vi "Dashboard Main.vi"() -> ()   [LabVIEW 2020]
uses:
  <vilib>/Utility/miscctls.llb/LVRowAndColumnTypeDef.ctl
  <vilib>/event_ctls.llb/eventvkey.ctl
  <vilib>/Rock Robotics/Network Tables/NT Read Boolean.vi
  <vilib>/Rock Robotics/WPI/Dashboard/WPI_DashboardLogging Global.vi
panel:
  in  "Camera Settings Right":T1={"Frame Rate"=30, "Compression"=30, "Size"=1, "DB Camera Config"=FALSE} {"Frame Rate" scale=1.0..30.0; "Compression" scale=100.0..-1.0; "Size" items=["640x480", "320x240", "160x120"]}
  in  "Camera Name Right":string(combo)="No Camera Selection"
  out "Camera Perf":string
  in  "Camera Settings":T1={"Frame Rate"=30, "Compression"=30, "Size"=1, "DB Camera Config"=FALSE} {"Frame Rate" scale=1.0..30.0; "Compression" scale=100.0..-1.0; "Size" items=["640x480", "320x240", "160x120"]}
  in  "TCP":refnum<k5>
  in  "Rec Mode":enum32{"Stop", "Record", "Playback"}(radio)
  out "Robot IP":string
  out "Image Message":string="Timeout in Camera Communications"
  in  "Dashboard Tab":T2(tab)
  out "Grabber Motor On\nOuttake":bool
  out "Grabber Motor On\nIntake":bool
  out "Grabber Tilt Encoder R":dbl
  out "Hall Effect High":bool
  out "Hall Effect Low":bool
  out "Elevator Encoder R":dbl
  out "Elevator Encoder L":dbl
  out "Backwards Drive\nOn":bool
  out "Slow Speed\nOn":bool
  in  "Select Auto":string(combo)="Select Autonomous ..."
  out "NT Connection":bool
  out "Gyro":dbl(knob) scale=0.0..360.0
  out "Mode":T3(ring)=enum."Auto Disabled"
  out "Right Camera Perf":cluster{"Bandwidth (Mbps)":dbl, "FPS":dbl}
  out "Camera Image Right":T4(plugin-control)
  in  "DB/String 9":string
  in  "DB/String 8":string
  in  "DB/String 7":string
  in  "DB/String 6":string
  in  "DB/String 5":string
  in  "DB/String 4":string
  in  "DB/String 3":string
  in  "DB/String 2":string
  in  "DB/String 1":string
  in  "DB/String 0":string
  in  "DB/Slider 0":dbl(slide) scale=0.0..5.0
  in  "DB/Slider 1":dbl(slide) scale=0.0..5.0
  in  "DB/Slider 2":dbl(slide) scale=0.0..5.0
  in  "DB/Slider 3":dbl(slide) scale=0.0..5.0
  out "DB/LED 3":bool
  out "DB/LED 2":bool
  out "DB/LED 1":bool
  out "DB/LED 0":bool
  in  "DB/Button 3":bool
  in  "DB/Button 2":bool
  in  "DB/Button 1":bool
  in  "DB/Button 0":bool caption="New Name"
  in  "Test Slider":dbl(slide) scale=0.0..100.0 scale format="%#_3g"
  in  "On/Off":bool caption="Solenoid"
  in  "Test Name":u16(ring) items=["Select the test to run..."]
  in  "Test Tree":string(tree)
  in  "Motor":cluster{"Value":dbl, "Enable":bool} {"Value" scale=-1.0..1.0 scale format="%#_3g"}
  out "Progress":T5 {"Test Progress" scale=0.0..100.0}
  in  "Rev/Fwd":cluster{"Forward":bool, "Reverse":bool}
  in  "Test Ring":u16(ring) items=["Monochrome", "Color"]
  out "Cmd Status":string
  in  "Execute Command":bool
  in  "Command Params":string[][](table)
  in  "Command Selection":i32(listbox)
  in  "CheckList":i32(listbox)
  out "Tree":string(tree)
  out "Camera Image":T4(plugin-control)
  out "Background":bool
  in  "Camera Name":string(combo)="No Camera Selection"
  # "HW"
  # "HW"
  # "This tab is a great place for autonomous settings and robot-specific values.\nPlace controls and indicators inside this tab and match name to\nDashboard Variables on robot. You can also delete this comment."
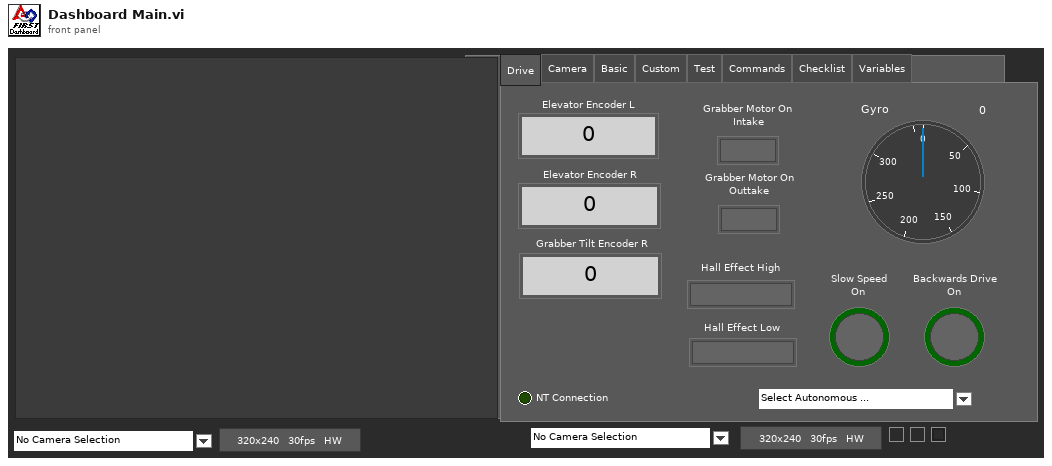
[diagram p1: front panel]
types:
  T1 = cluster{"Frame Rate":i32, "Compression":i32, "Size":u16, "DB Camera Config":bool}
  T2 = enum32{"Drive", "Camera", "Basic", "Custom", "Test", "Commands", "Checklist", "Variables"}
  T3 = enum8{"Tele-Op Disabled", "Tele-Op Enabled", "Auto Disabled", "Auto Enabled", "Test Disabled", "Test Enabled", "Disconnected", "No Code", "E-Stop"}
  T4 = typedef "IMAQ Image.ctl" = refnum<image>
  T5 = cluster{"Test Progress":u8, "Test Progress Text":string}
  T6 = cluster{"Save Path":path, "Interval (s)":dbl, "Keep":i32}
  T7 = typedef "Image Type" = u32
  T8 = cluster{"IDs":cluster{"RPC field ID":u16, "Unique ID":u16}, "String":string}
  T9 = cluster{"Error Strings":string, "Disable Counts":cluster{u16, u16}, "Rail Faults":cluster{u16, u16, u16}, "Robot IP":string, "DB Mode":u8, "Event Info":cluster{"Name":string, "Type":u8, "Number":u16, "Replay":u8}}
  T10 = cluster{"Storage":cluster{"Disk Free":u64, "RAM Block":u32, "RAM free":u32}, "CPU Utilization":cluster{"CPU % ISR":sgl, "CPU % Time Crit":sgl, "CPU % Timed Str":sgl, "CPU % High":sgl, "CPU % Above":sgl, "CPU % Normal":sgl, "CPU % Low":sgl}, "CAN":cluster{"% Bus Utilization":sgl, "Bus Off Cnt":u32, "TX_FIFO Full Cnt":u32, "Receive Error Cnt":u8, "Transmit Error Cnt":u8}, "HID":cluster{"HID Outputs":u32, "Rumble Low":u16, "Rumble High":u16}[]}
  T11 = cluster{"Status bits":cluster{"Test Mode":bool, "Autonomous":bool, "Enabled":bool, "Code Start":bool, "Brownout":bool, "Reserved 2":bool, "Reserved 3":bool, "E-Stop":bool}, "Code Trace":cluster{"Disabled":bool, "TeleOp":bool, "Auto":bool, "Test":bool}, "Controller Type":enum16{"unknown", "cRIO", "roboRio"}, "Code?":enum16{"unknown", "noCode", "code"}, "Battery V":dbl}
  T12 = cluster{"Control Bits":cluster{"TestMode":bool, "Autonomous":bool, "Enabled":bool, "FMS Present":bool, bool, bool, bool, "E-Stop":bool}, "Team Station ":u8, "Countdown":sgl, "Joystick Values":cluster{"Axes":dbl[], "Buttons":bool[], "POVs":i16[]}[]}
  T13 = cluster{"Camera Image":refnum<vi>, "Dashboard Tab":refnum<vi>, "Background":refnum<vi>, "Rec Mode":refnum<vi>, "Test Slider":refnum<vi>, "On/Off ":refnum<vi>, "Test Ring":refnum<vi>, "Rev/Fwd":refnum<vi>, "Test Name":refnum<vi>, "Motor":refnum<vi>, "Progress":refnum<vi>, "CheckList":refnum<vi>, "Tree":refnum<vi>, "Test Tree":refnum<vi>, "Command Params":refnum<vi>, "Command Selection":refnum<vi>, "Execute Command":refnum<vi>, "Cmd Status":refnum<vi>, "Camera Settings":refnum<vi>, "Camera Name":refnum<vi>, "Camera Perf":refnum<vi>, "Camera Settings Right":refnum<vi>, "Camera Name Right":refnum<vi>, "Camera Image Right":refnum<vi>}
  T14 = cluster{"Global Rectangle":i32[], "Contours":cluster{"Contour Type":u32, "ROI Type":u32, "Points":i32[]}[]}
  T15 = cluster{"Camera Name":string, string, "Saved DB Images Info":cluster{"Save Path":path, "Interval (s)":dbl, "Keep":i32}}
  T16 = cluster{"Camera Name Right":string, string, "Saved DB Images Info":cluster{"Save Path":path, "Interval (s)":dbl, "Keep":i32}}
  T17 = cluster{"Operation":enum16{"Update", "Clear"}, "Color Box":u32}[]
  T18 = typedef "eventvkey.ctl" = enum16{"ASCII", "Enter", "Return", "Shift", "Ctrl", "Alt", "Cmd", "Opt", "Caps", "NumLock", "Clear", "Break", "Up", "Down", "Left", "Right", "Insert", "Delete", "Home", "End", "PageUp", "PageDown", "Escape", "Help", "Pause", "ScrollLock", "F1", "F2", "F3", "F4", "F5", "F6", "F7", "F8", "F9", "F10", "F11", "F12", "F13", "F14", "F15", "F16", "F17", "F18", "F19", "F20", "F21", "F22", "F23", "F24", "Play", "VolumeUp", "VolumeDown", "Mute", "Two Byte Char"}
  T19 = cluster{"Image Size":bool, "Image Type":bool, "Pixel Value":bool, "ROI Information":bool, "Zoom Factor":bool}
  T20 = cluster{"Operation":enum16{"Update", "Clear"}, "Color Box":u32}
  T21 = typedef "LVRowAndColumnTypeDef.ctl" = cluster{"Row":i32, "Column":i32}
  T22 = cluster{"Shift":bool, "Ctrl":bool, "Alt":bool, "Cmd":bool, "Opt":bool}
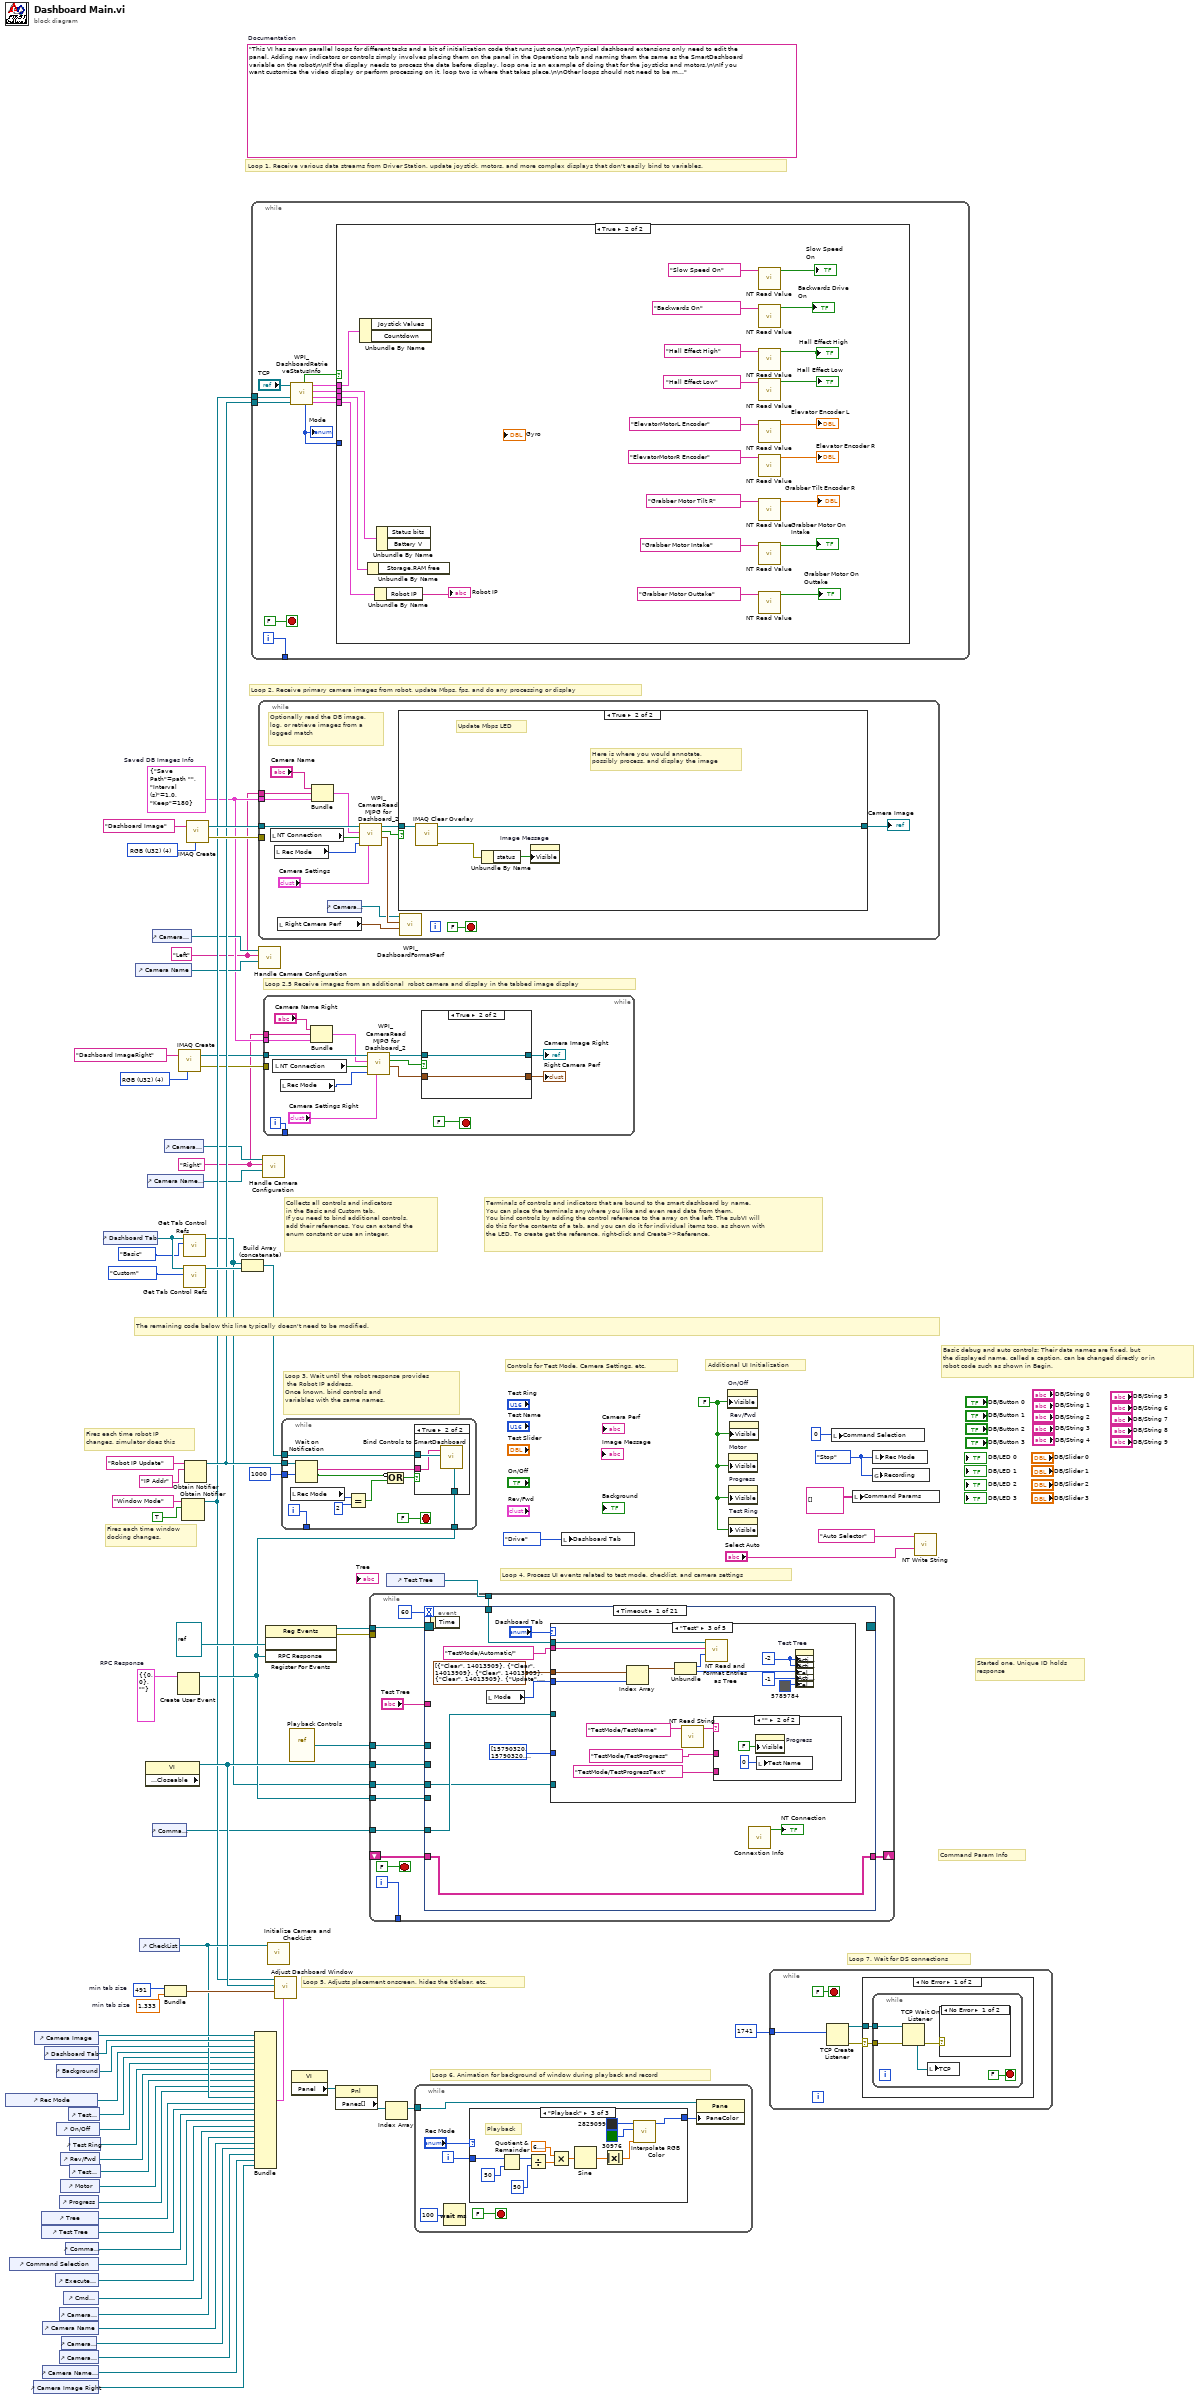
[diagram p0: block diagram]
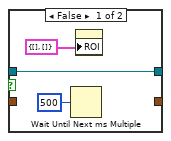
[diagram p2: hidden frame]
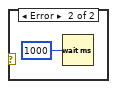
[diagram p3: hidden frame]
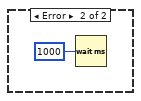
[diagram p4: hidden frame]
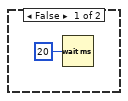
[diagram p5: hidden frame]
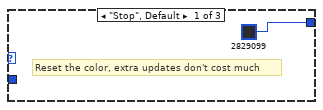
[diagram p6: hidden frame]
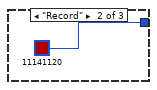
[diagram p7: hidden frame]
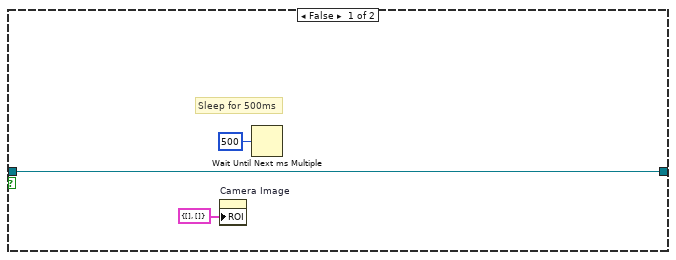
[diagram p9: hidden frame]
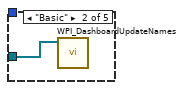
[diagram p11: hidden frame]
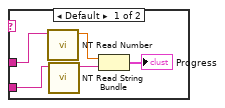
[diagram p12: hidden frame]
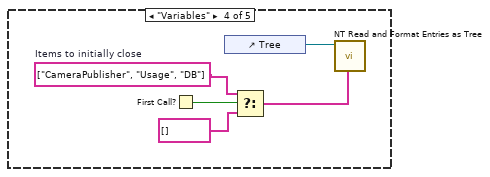
[diagram p13: hidden frame]
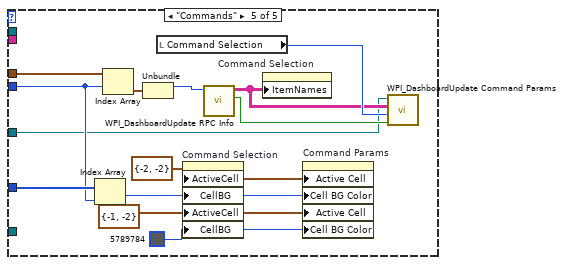
[diagram p14: hidden frame]
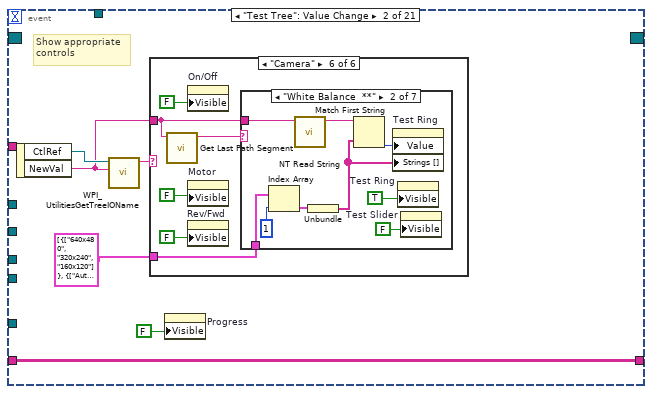
[diagram p15: hidden frame]
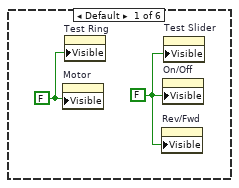
[diagram p16: hidden frame]
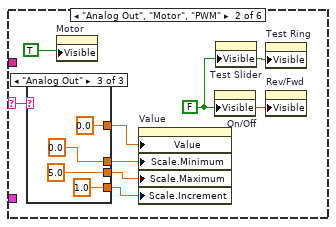
[diagram p17: hidden frame]
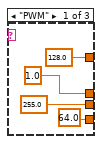
[diagram p18: hidden frame]
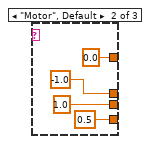
[diagram p19: hidden frame]
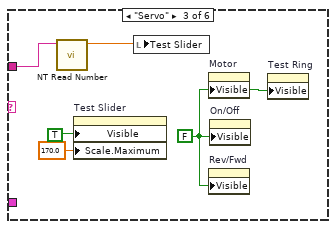
[diagram p20: hidden frame]
diagram:
  w3 = T6 {"Save Path"=path "", "Interval (s)"=1.0, "Keep"=180}  # Saved DB Images Info
  w2 = "Right"
  w1 = "Left"
  w13 = T7 4 items=["Grayscale (U8)", "Grayscale (I16)", "Grayscale (SGL)", "Complex (CSG)", "RGB (U32)", "HSL (U32)", "RGB (U64)"] ("Image Type")
  w29 = T8 {"IDs"={"RPC field ID"=0, "Unique ID"=0}, "String"=""}  # RPC Response
  w52 = 491  # min tab size
  w51 = 1.333  # min tab size
  w59 = enum32{"Stop", "Record", "Playback"}."Stop" ("Rec Mode")
  w36 = FALSE ("Visible")
  (unwired) "This VI has seven parallel loops for different tasks and a bit of initialization code that runs just once.\n\nTypical dashboard extensions only need to edit the panel. Adding new indicators or controls simply involves placing them on the panel in the Operations tab and naming them the same as the SmartDashboard variable on the robot\n\nIf the display needs to process the data before display, loop one is an example of doing that for the joysticks and motors.\n\nIf you want customize the video display or perform processing on it, loop two is where that takes place.\n\nOther loops should not need to be modified. They are pretty standard, and document the task they perform."  # Documentation
  w76 = T7 4 items=["Grayscale (U8)", "Grayscale (I16)", "Grayscale (SGL)", "Complex (CSG)", "RGB (U32)", "HSL (U32)", "RGB (U64)"] ("Image Type")
  # "Loop 2.5 Receive images from an additional  robot camera and display in the tabbed image display"
  # "Command Param Info"
  # "Started one, Unique ID holds\nresponse"
  # "Loop 7. Wait for DS connections"
  # "Basic debug and auto controls: Their data names are fixed, but\nthe displayed name, called a caption, can be changed directly or in\nrobot code such as shown in Begin."
  # "Controls for Test Mode, Camera Settings, etc."
  # "Additional UI Initialization"
  # "Loop 6. Animation for background of window during playback and record"
  # "Fires each time robot IP\nchanges, simulator does this"
  # "Fires each time window\ndocking changes."
  # "Collects all controls and indicators\nin the Basic and Custom tab.\nIf you need to bind additional controls,\nadd their references. You can extend the\nenum constant or use an integer."
  # "The remaining code below this line typically doesn't need to be modified."
  # "Loop 4. Process UI events related to test mode, checklist, and camera settings"
  # "Terminals of controls and indicators that are bound to the smart dashboard by name.\nYou can place the terminals anywhere you like and even read data from them.\nYou bind controls by adding the control reference to the array on the left. The subVI will\ndo this for the contents of a tab, and you can do it for individual items too, as shown with\nthe LED. To create get the reference, right-click and Create>>Reference."
  # "Loop 3. Wait until the robot response provides\n the Robot IP address.\nOnce known, bind controls and\nvariables with the same names."
  # "Loop 5. Adjusts placement onscreen, hides the titlebar, etc."
  # "Loop 1. Receive various data streams from Driver Station, update joystick, motors, and more complex displays that don't easily bind to variables."
  # "Loop 2. Receive primary camera images from robot, update Mbps, fps, and do any processing or display"
  n1 = control-ref of="Rec Mode"() -> (w42:refnum<vi>)
  n2 = control-ref of="Command Selection"() -> (w28:refnum<vi>)
  n3 = control-ref of="Camera Image Right"() -> (w6:refnum<vi>)
  n4 = control-ref of="Camera Image"() -> (w54:refnum<vi>)
  n5 = control-ref of="Tree"() -> (w46:refnum<vi>)
  n6 = control-ref of="Test Tree"() -> (w45:refnum<vi>)
  n7 = control-ref of="Camera Name"() -> (w19:refnum<vi>)
  n8 = control-ref of="Camera Name Right"() -> (w7:refnum<vi>)
  n9 = control-ref of="Dashboard Tab"() -> (w53:refnum<vi>)
  n10 = control-ref of="Execute Command"() -> (w30:refnum<vi>)
  n11 = control-ref of="Background"() -> (w49:refnum<vi>)
  n12 = control-ref of="On/Off"() -> (w40:refnum<vi>)
  n13 = control-ref of="Progress"() -> (w37:refnum<vi>)
  n14 = control-ref of="Camera Settings"() -> (w20:refnum<vi>)
  n15 = control-ref of="Camera Settings Right"() -> (w8:refnum<vi>)
  n16 = control-ref of="Rev/Fwd"() -> (w38:refnum<vi>)
  n17 = control-ref of="Motor"() -> (w43:refnum<vi>)
  n18 = control-ref of="Camera Perf"() -> (w18:refnum<vi>)
  n19 = control-ref of="Cmd Status"() -> (w24:refnum<vi>)
  n20 = control-ref of="Command Params"() -> (w31:refnum<vi>)
  n21 = control-ref of="Test Slider"() -> (w41:refnum<vi>)
  n22 = control-ref of="Test Ring"() -> (w39:refnum<vi>)
  n23 = control-ref of="Test Name"() -> (w44:refnum<vi>)
  n24 = control-ref of="Dashboard Tab"() -> (w57:refnum<vi>)
  n25 = control-ref of="Camera Name"() -> (w21:refnum<vi>)
  n26 = control-ref of="CheckList"() -> (w47:refnum<vi>)
  n27 = property class="VI" props=["Front Panel.Closeable"]() -> (reference out=w58:refnum<vi>)  [unwired: 2 in, 2 out]
  n28 = control-ref of="Camera Name Right"() -> (w9:refnum<vi>)
  n29 = control-ref of="Camera Settings"() -> (w22:refnum<vi>)
  n30 = control-ref of="Command Params"() -> (w23:refnum<vi>)
  n31 = control-ref of="Camera Settings Right"() -> (w10:refnum<vi>)
  n32 = Bundle("min tab size"=w52, "min tab size"=w51) -> (w50:cluster{"min tab size":i32, "min tab size":dbl})  [unwired: 1 in]
  n33 = Create User Event(user event datatype=w29) -> (user event=w25:refnum<user-event>)  [unwired: 1 in, 1 out]
  n34 = call "IMAQ Create"("Image Name"="Dashboard ImageRight", "Image Type"=w13) -> ("New Image"=w12:T4, "error out"=w11:errorcluster)  [unwired: 2 in, 1 out]
  n35 = Obtain Notifier(name (unnamed)="Window Mode", notification data type=TRUE) -> (notifier out=w34:refnum<notifier>)  [unwired: 2 in, 2 out]
  n36 = call <vilib>:"Get Tab Control Refs.vi"("Page Index"=T2."Basic" ("Dashboard Tab"), "TabControl in"=w57) -> ("ControlsOnPage"=w17:refnum<vi>[])  [unwired: 9 in]
  n37 = call <vilib>:"Get Tab Control Refs.vi"("Page Index"=T2."Custom" ("Dashboard Tab"), "TabControl in"=w57) -> ("ControlsOnPage"=w56:refnum<vi>[])  [unwired: 9 in]
  n38 = Obtain Notifier(name (unnamed)="Robot IP Update", notification data type="IP Addr" ("name (unnamed)")) -> (notifier out=w35:refnum<notifier>)  [unwired: 2 in, 2 out]
  n39 = call "IMAQ Create"("Image Name"="Dashboard Image", "Image Type"=w76) -> ("New Image"=w74:T4, "error out"=w73:errorcluster)  [unwired: 2 in, 1 out]
  n40 = Build Array (concatenate)(w17, w56) -> (w55:refnum<vi>[])
  n41 = while {
    tunnel: [w86] -> _
    tunnel: w35 -> [w80]
    tunnel: w34 -> [w77]
    i -> [w86]
    stop <- FALSE stop-if-true
    n42 = call <vilib>:"WPI_DashboardRetrieveStatusInfo.vi"("Binding Refnum"=w80, "Window Mode Notifier"=w77, "TCP Cnx"="TCP") -> ("Power and Errors"=w81:T9, "Robot Metrics"=w84:T10, "Status Info"=w85:T11, "Control Info"=w82:T12, "Robot Mode"=w79:T3, "Process?"=w83:bool)  [unwired: 3 in]
    "Mode" <- w79
    n43 = case shown="True" w83 {
      tunnel: w85 -> [_ w111]
      tunnel: w84 -> [_ w110]
      tunnel: w82 -> [_ w109]
      tunnel: w81 -> [_ w108]
      tunnel: w79 -> [_ _]
      frame False {
        n44 = Wait (ms)(milliseconds to wait=u32 20) -> ()  [unwired: 1 out]
      }
      frame True {
        n45 = Unbundle By Name(w109) -> ()  [unwired: 2 out]
        n46 = Unbundle By Name(w110) -> ()  [unwired: 1 out]
        n47 = Unbundle By Name(w108) -> ("Robot IP"=→"Robot IP":string)
        n48 = Unbundle By Name(w111) -> ()  [unwired: 2 out]
        n49 = call-poly <vilib>:"NT Read Value.vi"("Name"="Slow Speed On") -> ("Boolean"=→"Slow Speed\nOn":bool)  [unwired: 9 in, 1 out]
        n50 = call-poly <vilib>:"NT Read Value.vi"("Name"="Backwards On") -> ("Boolean"=→"Backwards Drive\nOn":bool)  [unwired: 9 in, 1 out]
        n51 = call-poly <vilib>:"NT Read Value.vi"("Name"="Hall Effect High") -> ("Boolean"=→"Hall Effect High":bool)  [unwired: 9 in, 1 out]
        n52 = call-poly <vilib>:"NT Read Value.vi"("Name"="Hall Effect Low") -> ("Boolean"=→"Hall Effect Low":bool)  [unwired: 9 in, 1 out]
        n53 = call-poly <vilib>:"NT Read Value.vi"("Name"="ElevatorMotorL Encoder") -> ("Numeric"=→"Elevator Encoder L":dbl)  [unwired: 9 in, 1 out]
        n54 = call-poly <vilib>:"NT Read Value.vi"("Name"="ElevatorMotorR Encoder") -> ("Numeric"=→"Elevator Encoder R":dbl)  [unwired: 9 in, 1 out]
        n55 = call-poly <vilib>:"NT Read Value.vi"("Name"="Grabber Motor Tilt R") -> ("Numeric"=→"Grabber Tilt Encoder R":dbl)  [unwired: 9 in, 1 out]
        n56 = call-poly <vilib>:"NT Read Value.vi"("Name"="Grabber Motor Intake") -> ("Boolean"=→"Grabber Motor On\nIntake":bool)  [unwired: 9 in, 1 out]
        n57 = call-poly <vilib>:"NT Read Value.vi"("Name"="Grabber Motor Outtake") -> ("Boolean"=→"Grabber Motor On\nOuttake":bool)  [unwired: 9 in, 1 out]
      }
    }
  }
  n58 = Bundle("Camera Image"=w54, "Dashboard Tab"=w53, "Background"=w49, "Rec Mode"=w42, "Test Slider"=w41, "On/Off"=w40, "Test Ring"=w39, "Rev/Fwd"=w38, "Test Name"=w44, "Motor"=w43, "Progress"=w37, "CheckList"=w47, "Tree"=w46, "Test Tree"=w45, "Command Params"=w31, "Command Selection"=w28, "Execute Command"=w30, "Cmd Status"=w24, "Camera Settings"=w20, "Camera Name"=w19, "Camera Perf"=w18, "Camera Settings Right"=w8, "Camera Name Right"=w7, "Camera Image Right"=w6) -> (w48:T13)  [unwired: 1 in]
  n59 = call "Handle Camera Configuration.vi"("CameraNameRef"=w21, "Display Name"=w1, "ClusterRef"=w22) -> ()  [unwired: 9 in]
  n60 = while {
    tunnel: w74 -> [w125]
    tunnel: w73 -> [_]
    tunnel: w3 -> [w118]
    tunnel: w1 -> [w115]
    stop <- FALSE stop-if-true
    # "Optionally read the DB image,\nlog, or retrieve images from a\nlogged match"
    n61 = local read "NT Connection"() -> (w119:bool)
    n62 = local read "Rec Mode"() -> (w122:enum32{"Stop", "Record", "Playback"})
    n63 = local read "Right Camera Perf"() -> (w113:cluster{"Bandwidth (Mbps)":dbl, "FPS":dbl})
    n64 = Bundle("Camera Name"="Camera Name", w115, "Saved DB Images Info"=w118) -> (w117:T15)  [unwired: 1 in]
    n65 = control-ref of="Camera Perf"() -> (w112:refnum<vi>)
    n66 = call <vilib>:"WPI_CameraRead MJPG for Dashboard_2.vi"("Camera Settings"="Camera Settings", "Rec Mode"=w122, "NT Connection"=w119, "Capture Info"=w117, "Image in"=w125) -> ("perf info"=w114:cluster{"Bandwidth (Mbps)":dbl, "fps":dbl}, "Active"=w123:bool, "Image\\ out"=w124:T4)  [unwired: 4 in]
    n67 = case shown="True" w123 {
      tunnel: w124 -> [w128 w131]
      tunnel: [w128 w130] -> w120
      frame False {
        # "Sleep for 500ms"
        n68 = property on="Camera Image" class="ImageControl"("ROI"=T14 {"Global Rectangle"=[], "Contours"=[]}) -> ()  [unwired: 2 in, 2 out]
        n69 = Wait Until Next ms Multiple(millisecond multiple=u32 500) -> ()  [unwired: 1 out]
      }
      frame True {
        # "Here is where you would annotate,\npossibly process, and display the image"
        # "Update Mbps LED"
        n70 = call "IMAQ Clear Overlay"("Image"=w131) -> ("error out"=w132:errorcluster, "Image Out"=w130:T4)  [unwired: 2 in, 7 out]
        n71 = Unbundle By Name(w132) -> ("status"=w133:bool)
        n72 = property on="Image Message" class="Str"("Visible"=w133) -> ()  [unwired: 2 in, 2 out]
      }
    }
    "Camera Image" <- w120
    n73 = call <vilib>:"WPI_DashboardFormatPerf.vi"("Right Camera Perf"=w113, "Performance"=w114, "String in"=w112) -> ()  [unwired: 9 in]
  }
  n74 = call "Handle Camera Configuration.vi"("CameraNameRef"=w9, "Display Name"=w2, "ClusterRef"=w10) -> ()  [unwired: 9 in]
  n75 = while {
    tunnel: w12 -> [w148]
    tunnel: w11 -> [_]
    tunnel: [w143] -> _
    tunnel: w3 -> [w139]
    tunnel: w2 -> [w136]
    i -> [w143]
    stop <- FALSE stop-if-true
    n76 = local read "NT Connection"() -> (w140:bool)
    n77 = local read "Rec Mode"() -> (w147:enum32{"Stop", "Record", "Playback"})
    n78 = Bundle("Camera Name Right"="Camera Name Right", w136, "Saved DB Images Info"=w139) -> (w138:T16)  [unwired: 1 in]
    n79 = call <vilib>:"WPI_CameraRead MJPG for Dashboard_2.vi"("Camera Settings"="Camera Settings Right", "Rec Mode"=w147, "NT Connection"=w140, "Capture Info"=w138, "Image in"=w148) -> ("perf info"=w134:cluster{"Bandwidth (Mbps)":dbl, "fps":dbl}, "Active"=w142:bool, "Image\\ out"=w145:T4)  [unwired: 4 in]
    n80 = case shown="True" w142 {
      tunnel: w145 -> [w150 w153]
      tunnel: [w150 w153] -> w141
      tunnel: [_ w152] -> w135
      tunnel: w134 -> [_ w152]
      frame False {
        n81 = Wait Until Next ms Multiple(millisecond multiple=u32 500) -> ()  [unwired: 1 out]
        n82 = property on="Camera Image Right" class="ImageControl"("ROI"=T14 {"Global Rectangle"=[], "Contours"=[]}) -> ()  [unwired: 2 in, 2 out]
      }
      frame True {
      }
    }
    "Camera Image Right" <- w141
    "Right Camera Perf" <- w135
  }
  n83 = register-events(refnum<vi> refnum, w25) -> (reference out=w63:refnum<event-registration>, error out=w62:errorcluster)  [unwired: 2 in]
  n84 = call "Initialize Camera and CheckList.vi"("ListBox in"=w47) -> ()  [unwired: 11 in]
  n85 = call "Adjust Dashboard Window.vi"("Sizing Refnums"=w48, "Size Constraints"=w50, "VI"=w58, "WIn Mode"=w34) -> ()  [unwired: 8 in]
  n86 = while {
    tunnel: w55 -> [w165]
    tunnel: w35 -> [w163]
    tunnel: [w161] -> _
    tunnel: u32 1000 ("milliseconds to wait") -> [w160]
    tunnel: w25 -> [w154]
    i -> [w161]
    stop <- FALSE stop-if-true
    n87 = local read "Rec Mode"() -> (w156:enum32{"Stop", "Record", "Playback"})
    n88 = Wait on Notification(notifier=w163, timeout in ms (-1)=w160) -> (notification=w162:string, timed out?=w158:bool)  [unwired: 2 in, 2 out]
    n89 = Equal?(x=w156, y=u16 2 ("Rec Mode")) -> (x = y?=w157:bool)
    n90 = Compound Arithmetic op=OR(invert w158, w157) -> (w159:bool)
    n91 = case shown="True" w159 {
      tunnel: w165 -> [_ w168]
      tunnel: w162 -> [_ w167]
      tunnel: w154 -> [_ w166]
      frame False {
      }
      frame True {
        n92 = call <vilib>:"Bind Controls to SmartDashboard.vi"("RPC ref"=w166, "Bound Control Refs"=w168, "Server IP Address"=w167) -> ()  [unwired: 9 in]
      }
    }
  }
  n93 = vi-ref "Playback Controls.vi"() -> (w64:refnum<vi>)
  n94 = property class="VI"() -> ("Panel"=w66:refnum<vi>)  [unwired: 2 in, 2 out]
  n95 = property class="Pnl"(reference=w66) -> ("Panes[]"=w67:refnum<vi>[])  [unwired: 1 in, 2 out]
  n96 = Index Array(array=w67) -> (element=w65:refnum<vi>)  [unwired: 1 in]
  n97 = control-ref of="Test Tree"() -> (w68:refnum<vi>)
  n98 = while {
    tunnel: [w178] -> _
    tunnel: w68 -> [w177]
    tunnel: w64 -> [w176]
    tunnel: w63 -> [w175]
    tunnel: w62 -> [_]
    tunnel: w58 -> [w174]
    tunnel: w25 -> [w173]
    tunnel: w23 -> [w172]
    shift-right: [w171] -> _
    shift-left: _ -> [w170]
    tunnel: w17 -> [w169]
    i -> [w178]
    stop <- FALSE stop-if-true
    n99 = event shown="[0] Timeout" {
      selector: w175 -> [_ _ _ _ _ _ _ _ _ _ _ _ _ _ _ _ _ _ _ _ _]
      dyn-events: [_ _ _ _ _ _ _ _ _ _ _ _ _ _ _ _ w438 _ _ _ _] -> _
      timeout: u32 60 ("milliseconds to wait") -> [_ _ _ _ _ _ _ _ _ _ _ _ _ _ _ _ _ _ _ _ _]
      tunnel: w177 -> [w190 _ _ _ _ _ _ _ _ _ _ _ _ _ _ _ _ _ _ _ _]
      tunnel: "Test Tree" -> [_ _ _ _ _ _ _ _ _ _ _ w405 w413 w415 w419 w427 _ _ _ _ _]
      tunnel: w176 -> [_ _ _ _ _ _ _ _ _ _ _ _ _ _ _ _ w440 _ w458 _ _]
      tunnel: w174 -> [_ _ _ _ _ _ _ _ _ _ _ _ _ _ _ _ w436 _ _ _ _]
      tunnel: w173 -> [_ _ _ _ _ _ _ _ _ _ _ _ _ _ _ _ w434 _ _ _ _]
      tunnel: w172 -> [w185 _ _ _ _ _ w356 _ _ _ _ _ _ _ _ _ _ _ _ _ _]
      tunnel: [w184 w233 w335 w340 w349 w353 w354 w363 w373 w380 w392 w404 w411 w414 w418 w426 w433 w453 w455 w459 w472] -> w171
      tunnel: w170 -> [w184 w233 w335 w340 w349 w353 w354 _ _ w380 w392 w404 w411 w414 w418 w426 w433 w453 w455 w459 w472]
      tunnel: w169 -> [w182 _ _ _ _ _ _ _ _ _ _ _ _ _ _ _ _ _ _ _ _]
      event Timeout {
        n100 = event-data() -> ()  [unwired: 1 in, 1 out]
        n101 = local read "Mode"() -> (w187:T3)
        n102 = case shown="\"Test\"" "Dashboard Tab" {
          tunnel: w190 -> [_ _ w206 _ _]
          tunnel: "TestMode/Automatic/" ("Name Pattern") -> [_ _ w205 _ _]
          tunnel: T17 [{"Operation"=enum."Clear", "Color Box"=14013909}, {"Operation"=enum."Clear", "Color Box"=14013909}, {"Operation"=enum."Clear", "Color Box"=14013909}, {"Operation"=enum."Clear", "Color Box"=14013909}, {"Operation"=enum."Update", "Color Box"=14013909}, {"Operation"=enum."Update", "Color Box"=16777215}, {"Operation"=enum."Clear", "Color Box"=14013909}, {"Operation"=enum."Clear", "Color Box"=14013909}, {"Operation"=enum."Clear", "Color Box"=14013909}] -> [_ _ w198 _ w226]
          tunnel: w187 -> [_ _ w197 _ w225]
          tunnel: u32[] [15790320, 15790320, 15790320, 15790320, 16777215, 16777215, 15790320, 15790320, 15790320] -> [_ _ _ _ w231]
          tunnel: w185 -> [_ _ _ _ w219]
          tunnel: w182 -> [_ w192 _ _ _]
          frame "Custom", Default {
          }
          frame "Basic" {
            n103 = call <vilib>:"WPI_DashboardUpdateNames.vi"("Controls on Tab"=w192) -> ()  [unwired: 11 in]
          }
          frame "Test" {
            w204 = -2 ("Active Item:Row Number")
            n104 = Index Array(array=w198, index=w197) -> (element=w199:T20)
            n105 = Unbundle(w199) -> ("Operation"=w200:enum16{"Update", "Clear"}, "Color Box"=w201:u32)
            n106 = call <vilib>:"NT Read String.vi"("Name"="TestMode/TestName") -> ("String"=w195:string)  [unwired: 9 in, 1 out]
            n107 = call <vilib>:"NT Read and Format Entries as Tree.vi"("Operation"=w200, "Name Pattern"=w205, "Tree Refnum"=w206) -> ()  [unwired: 7 in, 2 out]
            n108 = case shown="\"\"" w195 {
              tunnel: "TestMode/TestProgress" ("Name") -> [w208 _]
              tunnel: "TestMode/TestProgressText" ("Name") -> [w207 _]
              frame Default {
                n109 = call <vilib>:"NT Read Number.vi"("Name"=w208) -> ("Numeric"=w209:dbl)  [unwired: 9 in, 1 out]
                n110 = call <vilib>:"NT Read String.vi"("Name"=w207) -> ("String"=w210:string)  [unwired: 9 in, 1 out]
                n111 = Bundle("Numeric"=w209, "String"=w210) -> (→"Progress":cluster{"Numeric":dbl, "String":string})  [unwired: 1 in]
              }
              frame "" {
                n112 = property on="Progress" class="Clust (strict)"("Visible"=FALSE) -> ()  [unwired: 2 in, 2 out]
                n113 = local write "Test Name"(u16 0) -> ()
              }
            }
            n114 = property on="Test Tree" class="Tree (strict)"("Active Item Row Number"=w204, "ActiveColNum"=w204, "CellBG"=w201, "Active Item Row Number"=-1 ("Active Item:Row Number"), "CellBG"=u32 5789784 ("Color Box")) -> ()  [unwired: 2 in, 2 out]
          }
          frame "Variables" {
            w216 = string[] ["CameraPublisher", "Usage", "DB"]  # Items to initially close
            n115 = First Call?() -> (First Call?: T/F=w217:bool)
            n116 = control-ref of="Tree"() -> (w218:refnum<vi>)
            n117 = Select(t=w216, s=w217, f=string[] []) -> (s? t:f=w214:string[])
            n118 = call <vilib>:"NT Read and Format Entries as Tree.vi"("Tags to  Close"=w214, "Tree Refnum"=w218) -> ()  [unwired: 8 in, 2 out]
          }
          frame "Commands" {
            w227 = u32 5789784 ("Color Box")
            w228 = T21 {"Row"=-1, "Column"=-2} ("Active Cell:Active Cell")
            w230 = T21 {"Row"=-2, "Column"=-2} ("Active Cell:Active Cell")
            n119 = Index Array(array=w231, index=w225) -> (element=w229:u32)
            n120 = Index Array(array=w226, index=w225) -> (element=w224:T20)
            n121 = Unbundle(w224) -> ("Operation"=w223:enum16{"Update", "Clear"})  [unwired: 1 out]
            n122 = local read "Command Selection"() -> (w222:i32)
            n123 = property on="Command Selection" class="MCListbox (strict)"("ActiveCell"=w230, "CellBG"=w229, "ActiveCell"=w228, "CellBG"=w227) -> ()  [unwired: 2 in, 2 out]
            n124 = call <vilib>:"WPI_DashboardUpdate RPC Info.vi"("Operation"=w223) -> ("update"=w221:bool, "commands"=w220:string[][])  [unwired: 9 in]
            n125 = property on="Command Selection" class="MCListbox (strict)"("ItemNames"=w220) -> ()  [unwired: 2 in, 2 out]
            n126 = property on="Command Params" class="Tbl (strict)"("Active Cell"=w230, "Cell BG Color"=w229, "Active Cell"=w228, "Cell BG Color"=w227) -> ()  [unwired: 2 in, 2 out]
            n127 = call <vilib>:"WPI_DashboardUpdate Command Params.vi"("Update"=w221, "NewVal"=w222, "Commands"=w220, "Param Tbl"=w219) -> ()  [unwired: 7 in, 1 out]
          }
        }
        n128 = call <vilib>:"Connextion Info.vi"() -> ("Connected"=→"NT Connection":bool)  [unwired: 10 in, 1 out]
      }
      event "Test Tree": Value Change {
        # "Show appropriate\ncontrols"
        n129 = event-data() -> ("CtlRef"=w236:refnum<vi>, "NewVal"=w234:string)  [unwired: 1 in]
        n130 = call <vilib>:"WPI_UtilitiesGetTreeIOName.vi"("NewVal"=w234, "TreeControl in"=w236) -> ("I/O Name"=w237:string)  [unwired: 9 in]
        n131 = case shown="\"Camera\"" w237 {
          selector: w237 -> [_ w244 _ w266 w275 _]
          tunnel: w234 -> [_ _ w263 w265 _ w282]
          tunnel: cluster{string[]}[] [{["640x480", "320x240", "160x120"]}, {["Auto", "Fixed indoor", "Fixed outdoor 1", "Fixed outdoor 2", "Fixed fluorescent 1", "Fixed fluorescent 2", "Hold current"]}, {["Auto", "Flicker-free 50 Hz", "Flicker-free 60 Hz", "Hold current"]}, {["None", "Prioritize frame rate", "Prioritize image quality"]}, {["Monochrome", "Color"]}] -> [_ _ _ _ _ w281]
          frame Default {
            w239 = FALSE ("Visible")
            w238 = FALSE ("Visible")
            n132 = property on="Motor" class="Clust (strict)"("Visible"=w238) -> ()  [unwired: 2 in, 2 out]
            n133 = property on="Test Ring" class="Ring (strict)"("Visible"=w238) -> ()  [unwired: 2 in, 2 out]
            n134 = property on="Rev/Fwd" class="Clust (strict)"("Visible"=w239) -> ()  [unwired: 2 in, 2 out]
            n135 = property on="On/Off" class="Bool (strict)"("Visible"=w239) -> ()  [unwired: 2 in, 2 out]
            n136 = property on="Test Slider" class="Slide (strict)"("Visible"=w239) -> ()  [unwired: 2 in, 2 out]
          }
          frame "Analog Out", "Motor", "PWM" {
            w245 = FALSE ("Visible")
            n137 = case shown="\"Analog Out\"" w244 {
              tunnel: [1.0 ("Value") -1.0 ("Value") 0.0 ("Value")] -> w243
              tunnel: [255.0 ("Value") 1.0 ("Value") 5.0 ("Value")] -> w242
              tunnel: [128.0 ("Value") 0.0 ("Value") 0.0 ("Value")] -> w241
              tunnel: [64.0 ("Value") 0.5 ("Value") 1.0 ("Value")] -> w240
              frame "PWM" {
              }
              frame "Motor", Default {
              }
              frame "Analog Out" {
              }
            }
            n138 = property on="Motor" class="Clust (strict)"("Visible"=TRUE) -> ()  [unwired: 2 in, 2 out]
            n139 = property on="Value" class="Slide (strict)"("Value"=w241, "Scale.Minimum"=w243, "Scale.Maximum"=w242, "Scale.Increment"=w240) -> ()  [unwired: 2 in, 2 out]
            n140 = property on="On/Off" class="Bool (strict)"("Visible"=w245) -> ()  [unwired: 2 in, 2 out]
            n141 = property on="Test Slider" class="Slide (strict)"("Visible"=w245) -> ()  [unwired: 2 in, 2 out]
            n142 = property on="Test Ring" class="Ring (strict)"("Visible"=w245) -> ()  [unwired: 2 in, 2 out]
            n143 = property on="Rev/Fwd" class="Clust (strict)"("Visible"=w245) -> ()  [unwired: 2 in, 2 out]
          }
          frame "Servo" {
            w261 = FALSE ("Visible")
            n144 = call <vilib>:"NT Read Number.vi"("Name"=w263) -> ("Numeric"=w262:dbl)  [unwired: 9 in, 1 out]
            n145 = property on="Test Slider" class="Slide (strict)"("Visible"=TRUE, "Scale.Maximum"=170.0 ("Scale.Range:Maximum")) -> ()  [unwired: 2 in, 2 out]
            n146 = local write "Test Slider"(w262) -> ()
            n147 = property on="Motor" class="Clust (strict)"("Visible"=w261) -> ()  [unwired: 2 in, 2 out]
            n148 = property on="Rev/Fwd" class="Clust (strict)"("Visible"=w261) -> ()  [unwired: 2 in, 2 out]
            n149 = property on="On/Off" class="Bool (strict)"("Visible"=w261) -> ()  [unwired: 2 in, 2 out]
            n150 = property on="Test Ring" class="Ring (strict)"("Visible"=w261) -> ()  [unwired: 2 in, 2 out]
          }
          frame "Relay", "Solenoid" {
            w264 = FALSE ("Visible")
            n151 = property on="Motor" class="Clust (strict)"("Visible"=w264) -> ()  [unwired: 2 in, 2 out]
            n152 = property on="Test Slider" class="Slide (strict)"("Visible"=w264) -> ()  [unwired: 2 in, 2 out]
            n153 = Search and Replace String(input string=w265, search string="/Value  **", replace string="/Direction") -> (result string=w271:string)  [unwired: 5 in, 3 out]
            n154 = property on="Test Ring" class="Ring (strict)"("Visible"=w264) -> ()  [unwired: 2 in, 2 out]
            n155 = call <vilib>:"NT Read String.vi"("Name"=w271) -> ("String"=w269:string)  [unwired: 9 in, 1 out]
            n156 = Equal?(x="Both directions", y=w269) -> (x = y?=w267:bool)
            n157 = Not(x=w267) -> (.not. x?=w268:bool)
            n158 = property on="Rev/Fwd" class="Clust (strict)"("Visible"=w267) -> ()  [unwired: 2 in, 2 out]
            n159 = property on="On/Off" class="Bool (strict)"("Visible"=w268, "Caption.Text"=w266) -> ()  [unwired: 2 in, 2 out]
          }
          frame "Compressor", "Digital Out" {
            w274 = FALSE ("Visible")
            # "Get direction and finish"
            n160 = property on="Motor" class="Clust (strict)"("Visible"=w274) -> ()  [unwired: 2 in, 2 out]
            n161 = property on="Test Slider" class="Slide (strict)"("Visible"=w274) -> ()  [unwired: 2 in, 2 out]
            n162 = property on="Test Ring" class="Ring (strict)"("Visible"=w274) -> ()  [unwired: 2 in, 2 out]
            n163 = property on="On/Off" class="Bool (strict)"("Visible"=TRUE, "Caption.Text"=w275) -> ()  [unwired: 2 in, 2 out]
            n164 = property on="Rev/Fwd" class="Clust (strict)"("Visible"=FALSE) -> ()  [unwired: 2 in, 2 out]
          }
          frame "Camera" {
            n165 = call <vilib>:"Get Last Path Segment.vi"("String in"=w282) -> ("String out"=w283:string)  [unwired: 10 in]
            n166 = property on="On/Off" class="Bool (strict)"("Visible"=FALSE) -> ()  [unwired: 2 in, 2 out]
            n167 = property on="Motor" class="Clust (strict)"("Visible"=FALSE) -> ()  [unwired: 2 in, 2 out]
            n168 = property on="Rev/Fwd" class="Clust (strict)"("Visible"=FALSE) -> ()  [unwired: 2 in, 2 out]
            n169 = case shown="\"White Balance  **\"" w283 {
              tunnel: w282 -> [w289 w298 w307 w316 w325 _ w331]
              tunnel: w281 -> [w287 w295 w304 w313 w322 _ _]
              frame "Size  **" {
                n170 = Index Array(array=w287) -> (element=w286:cluster{string[]})  [unwired: 1 in]
                n171 = call <vilib>:"NT Read String.vi"("Name"=w289) -> ("String"=w288:string)  [unwired: 9 in, 1 out]
                n172 = Unbundle(w286) -> (w284:string[])
                n173 = Match First String(2:w284, 3:w288) -> (0:w285:i32)  [unwired: 1 out]
                n174 = property on="Test Ring" class="Ring (strict)"("Value"=w285, "Strings []"=w284) -> ()  [unwired: 2 in, 2 out]
                n175 = property on="Test Ring" class="Ring (strict)"("Visible"=TRUE) -> ()  [unwired: 2 in, 2 out]
                n176 = property on="Test Slider" class="Slide (strict)"("Visible"=FALSE) -> ()  [unwired: 2 in, 2 out]
              }
              frame "White Balance  **" {
                n177 = Index Array(array=w295, index=1) -> (element=w296:cluster{string[]})
                n178 = call <vilib>:"NT Read String.vi"("Name"=w298) -> ("String"=w297:string)  [unwired: 9 in, 1 out]
                n179 = Unbundle(w296) -> (w293:string[])
                n180 = Match First String(2:w293, 3:w297) -> (0:w292:i32)  [unwired: 1 out]
                n181 = property on="Test Ring" class="Ring (strict)"("Value"=w292, "Strings []"=w293) -> ()  [unwired: 2 in, 2 out]
                n182 = property on="Test Ring" class="Ring (strict)"("Visible"=TRUE) -> ()  [unwired: 2 in, 2 out]
                n183 = property on="Test Slider" class="Slide (strict)"("Visible"=FALSE) -> ()  [unwired: 2 in, 2 out]
              }
              frame "Exposure  **" {
                n184 = Index Array(array=w304, index=2) -> (element=w305:cluster{string[]})
                n185 = call <vilib>:"NT Read String.vi"("Name"=w307) -> ("String"=w306:string)  [unwired: 9 in, 1 out]
                n186 = Unbundle(w305) -> (w301:string[])
                n187 = Match First String(2:w301, 3:w306) -> (0:w302:i32)  [unwired: 1 out]
                n188 = property on="Test Ring" class="Ring (strict)"("Value"=w302, "Strings []"=w301) -> ()  [unwired: 2 in, 2 out]
                n189 = property on="Test Ring" class="Ring (strict)"("Visible"=TRUE) -> ()  [unwired: 2 in, 2 out]
                n190 = property on="Test Slider" class="Slide (strict)"("Visible"=FALSE) -> ()  [unwired: 2 in, 2 out]
              }
              frame "Exposure Priority  **" {
                n191 = Index Array(array=w313, index=3) -> (element=w314:cluster{string[]})
                n192 = call <vilib>:"NT Read String.vi"("Name"=w316) -> ("String"=w315:string)  [unwired: 9 in, 1 out]
                n193 = Unbundle(w314) -> (w310:string[])
                n194 = Match First String(2:w310, 3:w315) -> (0:w311:i32)  [unwired: 1 out]
                n195 = property on="Test Ring" class="Ring (strict)"("Value"=w311, "Strings []"=w310) -> ()  [unwired: 2 in, 2 out]
                n196 = property on="Test Ring" class="Ring (strict)"("Visible"=TRUE) -> ()  [unwired: 2 in, 2 out]
                n197 = property on="Test Slider" class="Slide (strict)"("Visible"=FALSE) -> ()  [unwired: 2 in, 2 out]
              }
              frame "Color Enable  **" {
                n198 = Index Array(array=w322, index=4) -> (element=w323:cluster{string[]})
                n199 = call <vilib>:"NT Read String.vi"("Name"=w325) -> ("String"=w324:string)  [unwired: 9 in, 1 out]
                n200 = Unbundle(w323) -> (w319:string[])
                n201 = Match First String(2:w319, 3:w324) -> (0:w320:i32)  [unwired: 1 out]
                n202 = property on="Test Ring" class="Ring (strict)"("Value"=w320, "Strings []"=w319) -> ()  [unwired: 2 in, 2 out]
                n203 = property on="Test Ring" class="Ring (strict)"("Visible"=TRUE) -> ()  [unwired: 2 in, 2 out]
                n204 = property on="Test Slider" class="Slide (strict)"("Visible"=FALSE) -> ()  [unwired: 2 in, 2 out]
              }
              frame Default {
                n205 = property on="Test Ring" class="Ring (strict)"("Visible"=FALSE) -> ()  [unwired: 2 in, 2 out]
                n206 = property on="Test Slider" class="Slide (strict)"("Visible"=FALSE) -> ()  [unwired: 2 in, 2 out]
              }
              frame "Brightness  **", "Color Level  **", "Compression  **", "FPS  **", "Sharpness  **" {
                n207 = call <vilib>:"NT Read Number.vi"("Name"=w331) -> ("Numeric"=w330:dbl)  [unwired: 9 in, 1 out]
                n208 = local write "Test Slider"(w330) -> ()
                n209 = property on="Test Slider" class="Slide (strict)"("Visible"=TRUE, "Scale.Maximum"=100.0 ("Scale.Range:Maximum")) -> ()  [unwired: 2 in, 2 out]
                n210 = property on="Test Ring" class="Ring (strict)"("Visible"=FALSE) -> ()  [unwired: 2 in, 2 out]
              }
            }
          }
        }
        n211 = property on="Progress" class="Clust (strict)"("Visible"=FALSE) -> ()  [unwired: 2 in, 2 out]
      }
      event "Test Name": Mouse Enter {
        # "Populate the ring with the list of tests"
        n212 = event-data() -> ()  [unwired: 1 in, 1 out]
        n213 = call <vilib>:"NT Read String Array.vi"("Name"="TestMode/TestList") -> ("String Array"=w339:string[])  [unwired: 9 in, 1 out]
        n214 = Build Array (concatenate)("Select the test to run...", w339) -> (w338:string[])
        n215 = property on="Test Name" class="Ring (strict)"("Strings []"=w338) -> ()  [unwired: 2 in, 2 out]
      }
      event "Test Name": Value Change {
        w341 = FALSE ("Visible")
        # "Tell the robot the test name to run"
        n216 = event-data() -> ("NewVal"=w345:u16)  [unwired: 1 in]
        n217 = property on="Test Name" class="Ring (strict)"() -> ("Strings []"=w346:string[])  [unwired: 2 in, 2 out]
        n218 = local write "Progress"(T5 {"Test Progress"=0, "Test Progress Text"=""} ("Progress")) -> ()
        n219 = Index Array(array=w346, index=w345) -> (element=w344:string)
        n220 = call <vilib>:"NT Write String.vi"("String"=w344, "Name"="TestMode/TestName") -> ()  [unwired: 9 in, 1 out]
        n221 = property on="Progress" class="Clust (strict)"("Visible"=TRUE) -> ()  [unwired: 2 in, 2 out]
        n222 = property on="Motor" class="Clust (strict)"("Visible"=w341) -> ()  [unwired: 2 in, 2 out]
        n223 = property on="Test Slider" class="Slide (strict)"("Visible"=w341) -> ()  [unwired: 2 in, 2 out]
        n224 = property on="On/Off" class="Bool (strict)"("Visible"=w341) -> ()  [unwired: 2 in, 2 out]
        n225 = property on="Rev/Fwd" class="Clust (strict)"("Visible"=w341) -> ()  [unwired: 2 in, 2 out]
        n226 = property on="Test Ring" class="Ring (strict)"("Visible"=w341) -> ()  [unwired: 2 in, 2 out]
      }
      event "Select Auto": Mouse Enter {
        # "Populate the combo box with the list of autonomous options"
        n227 = event-data() -> ()  [unwired: 1 in, 1 out]
        n228 = call <vilib>:"NT Read String Array.vi"("Name"="Auto List") -> ("String Array"=w348:string[])  [unwired: 9 in, 1 out]
        n229 = property on="Select Auto" class="CmbBox"("Strings[]"=w348) -> ()  [unwired: 2 in, 2 out]
      }
      event "Select Auto": Value Change {
        # "User modified the Auto Selection. Write to NT variable so robot knows."
        n230 = event-data() -> ("NewVal"=w351:string)  [unwired: 1 in]
        n231 = call <vilib>:"NT Write String.vi"("String"=w351, "Name"="Auto Selector") -> ()  [unwired: 9 in, 1 out]
      }
      event "Command Selection": Value Change {
        # "Get the params and show in table"
        n232 = event-data() -> ("NewVal"=w357:i32)  [unwired: 1 in]
        n233 = property on="Command Selection" class="MCListbox (strict)"() -> ("ItemNames"=w355:string[][])  [unwired: 2 in, 2 out]
        n234 = call <vilib>:"WPI_DashboardUpdate Command Params.vi"("NewVal"=w357, "Commands"=w355, "Param Tbl"=w356) -> ()  [unwired: 8 in, 1 out]
      }
      event "Execute Command": Value Change {
        # "Started one, Unique ID holds\nresponse"
        n235 = event-data() -> ()  [unwired: 1 in, 1 out]
        n236 = property on="Command Selection" class="MCListbox (strict)"() -> ("ItemNames"=w368:string[][])  [unwired: 2 in, 2 out]
        n237 = Index Array(array=w368, index (row)="Command Selection", index (col)=0) -> (element=w366:string)
        n238 = call <vilib>:"Invoke Commands.vi"("Command Params"="Command Params", "Function Name"=w366) -> ("Params"=w362:u8, "Started"=w361:bool)  [unwired: 7 in, 1 out]
        n239 = Array Subset(array="Command Params", length (row)=w362) -> (w363:string[][])  [unwired: 3 in]
        n240 = Select(t="Executing" ("Cmd Status"), s=w361, f="" ("Cmd Status")) -> (s? t:f=→"Cmd Status":string)
      }
      event "Command Selection": Double Click {
        n241 = event-data() -> ("Row"=w376:i32)  [unwired: 1 in]
        n242 = property on="Command Selection" class="MCListbox (strict)"() -> ("ItemNames"=w379:string[][])  [unwired: 2 in, 2 out]
        n243 = local read "Command Params"() -> (w375:string[][])
        n244 = Index Array(array=w379, index (row)=w376, index (col)=0) -> (element=w377:string)
        n245 = call <vilib>:"Invoke Commands.vi"("Command Params"=w375, "Function Name"=w377) -> ("Params"=w374:u8, "Started"=w369:bool)  [unwired: 7 in, 1 out]
        n246 = Array Subset(array=w375, length (row)=w374) -> (w373:string[][])  [unwired: 3 in]
        n247 = Select(t="Executing" ("Cmd Status"), s=w369, f="" ("Cmd Status")) -> (s? t:f=w370:string)
        n248 = local write "Cmd Status"(w370) -> ()
      }
      event "CheckList": Double Click {
        # "Shift clears all"
        # "Update symbols on the listbox"
        n249 = event-data() -> ("PlatMods.Shift"=w381:bool, "Row"=w383:i32)  [unwired: 1 in]
        n250 = case shown="True" w381 {
          tunnel: w383 -> [w387 _]
          tunnel: 1 -> [w386 _]
          frame False {
            n251 = property on="CheckList" class="LstBox (strict)"() -> ("Item Symbols"=w385:i32[])  [unwired: 2 in, 2 out]
            n252 = Replace Array Subset(array=w385, new element=w386, index=w387) -> (w384:i32[])
            n253 = property on="CheckList" class="LstBox (strict)"("Item Symbols"=w384) -> ()  [unwired: 2 in, 2 out]
          }
          frame True {
            w388 = 0 ("Top Row")
            n254 = property on="CheckList" class="LstBox (strict)"() -> ("Number of Rows"=w390:u32)  [unwired: 2 in, 2 out]
            n255 = Initialize Array(0, w390) -> (w389:i32[])
            n256 = property on="CheckList" class="LstBox (strict)"("Top Row"=w388, "Value"=w388, "Item Symbols"=w389) -> ()  [unwired: 2 in, 2 out]
          }
        }
      }
      event "CheckList": Key Down {
        # "Update symbols on the listbox\nLeft and right keys check and uncheck"
        n257 = event-data() -> ("VKey"=w394:T18)  [unwired: 1 in]
        n258 = case shown="\"Left\", \"Right\"" w394 {
          selector: w394 -> [w399 _]
          tunnel: eventvkey."Left" ("VKey") -> [w397 _]
          frame "Left", "Right" {
            n259 = Equal?(x=w397, y=w399) -> (x = y?=w398:bool)
            n260 = Select(t=0, s=w398, f=1) -> (s? t:f=w400:i32)
            n261 = property on="CheckList" class="LstBox (strict)"() -> ("Item Symbols"=w403:i32[])  [unwired: 2 in, 2 out]
            n262 = Replace Array Subset(array=w403, new element=w400, index="CheckList") -> (w402:i32[])
            n263 = property on="CheckList" class="LstBox (strict)"("Item Symbols"=w402) -> ()  [unwired: 2 in, 2 out]
          }
          frame Default {
          }
        }
      }
      event "Motor.Enable": Value Change {
        # "When the test mode otor enable helper is set, update that\ntree row item's value"
        n264 = event-data() -> ("NewVal"=w409:bool)  [unwired: 1 in]
        n265 = Unbundle("Motor") -> ("Value"=w408:dbl)  [unwired: 1 out]
        n266 = Select(t=w408, s=w409, f=0.0) -> (s? t:f=w406:dbl)
        n267 = call <vilib>:"NT Write Number.vi"("Numeric"=w406, "Name"=w405) -> ()  [unwired: 9 in, 1 out]
      }
      event "Test Slider": Value Change {
        # "When the test mode slider helper is set, update that\ntree row item's value"
        n268 = event-data() -> ("NewVal"=w412:dbl)  [unwired: 1 in]
        n269 = call <vilib>:"NT Write Number.vi"("Numeric"=w412, "Name"=w413) -> ()  [unwired: 9 in, 1 out]
      }
      event "On/Off": Value Change {
        # "When the test mode on/off helper value is set, update that\ntree row item's value"
        n270 = event-data() -> ("NewVal"=w417:bool)  [unwired: 1 in]
        n271 = Boolean To (0,1)(Boolean=w417) -> (0, 1=w416:i16)
        n272 = call <vilib>:"NT Write Number.vi"("Numeric"=w416, "Name"=w415) -> ()  [unwired: 9 in, 1 out]
      }
      event "Rev/Fwd": Value Change {
        # "When the test mode helper value for relays is set, update that\ntree row item's value"
        n273 = event-data() -> ("NewVal.Forward"=w425:bool, "NewVal.Reverse"=w424:bool)  [unwired: 1 in]
        n274 = Boolean To (0,1)(Boolean=w425) -> (0, 1=w421:i16)
        n275 = Boolean To (0,1)(Boolean=w424) -> (0, 1=w423:i16)
        n276 = Negate(x=w423) -> (-x=w422:i16)
        n277 = Add(x=w421, y=w422) -> (x+y=w420:i16)
        n278 = call <vilib>:"NT Write Number.vi"("Numeric"=w420, "Name"=w419) -> ()  [unwired: 9 in, 1 out]
      }
      event "Test Ring": Value Change {
        # "When a test mode helper value is selected from the ring,\nset the tree item's variable to the string value"
        n279 = event-data() -> ("NewVal"=w429:u16)  [unwired: 1 in]
        n280 = property on="Test Ring" class="Ring (strict)"() -> ("Strings []"=w430:string[])  [unwired: 2 in, 2 out]
        n281 = Index Array(array=w430, index=w429) -> (element=w428:string)
        n282 = call <vilib>:"NT Write String.vi"("String"=w428, "Name"=w427) -> ()  [unwired: 9 in, 1 out]
      }
      event "Rec Mode": Value Change {
        # "Update globals for recording mode and path to read log from.\nClear when logging and let NetworkTables set path for vision to\nuse."
        n283 = event-data() -> ("NewVal"=w441:enum32{"Stop", "Record", "Playback"})  [unwired: 1 in]
        n284 = global write "WPI_DashboardLogging Global.vi" "Logging Filename"(path "") -> ()
        n285 = global write "WPI_DashboardLogging Global.vi" "Recording"(w441) -> ()
        n286 = case shown="\"Playback\"" w441 {
          tunnel: w440 -> [_ w443 w452]
          tunnel: [_ _ w451] -> w438
          tunnel: [_ _ w450] -> _
          tunnel: w436 -> [_ _ w448]
          tunnel: cluster{i32, i32} {-250, 170} -> [_ _ w447]
          tunnel: [_ _ T19 {"Image Size"=TRUE, "Image Type"=TRUE, "Pixel Value"=TRUE, "ROI Information"=TRUE, "Zoom Factor"=FALSE} ("Image Information Shown:All Elements")] -> w431
          tunnel: [_ _ TRUE ("Zoom Factor")] -> w432
          tunnel: w434 -> [_ _ w444]
          frame Default {
          }
          frame "Stop", "Record" {
            # "Place Window too"
            n287 = invoke class="VI" method="FP.Close"(reference=w443) -> (reference out=w442:refnum<vi>)  [unwired: 2 in, 2 out]
            n288 = invoke class="VI" method="Abort VI"(reference=w442) -> ()  [unwired: 2 in, 3 out]
          }
          frame "Playback" {
            n289 = call "Open Playback Panel.vi"("Offset"=w447, "DB VI Ref"=w448, "Playback in"=w452) -> ("Playback out"=w449:refnum<vi>)  [unwired: 8 in]
            n290 = register-events(w449, w444) -> (reference out=w451:refnum<event-registration>, error out=w450:errorcluster)  [unwired: 2 in]
          }
        }
        n291 = property on="Camera Image Right" class="ImageControl"("Image Information Shown"=w431, "Image Information Visible"=w432) -> ()  [unwired: 2 in, 2 out]
        n292 = property on="Camera Image" class="ImageControl"("Image Information Shown"=w431, "Image Information Visible"=w432) -> ()  [unwired: 2 in, 2 out]
        n293 = call <vilib>:"WPI_DashboardNT Log FieldName Cache.vi"("Operation"=enum16{"Lookup/Add", "Index", "Clear"}."Clear") -> ()  [unwired: 8 in, 3 out]
      }
      event Panel Close {
        w454 = enum32{"Stop", "Record", "Playback"}."Stop" ("Rec Mode")
        # "Playback window has been closed, abort"
        n294 = event-data() -> ()  [unwired: 1 in, 4 out]
        n295 = local write "Rec Mode"(w454) -> ()
        n296 = global write "WPI_DashboardLogging Global.vi" "Recording"(w454) -> ()
      }
      event Panel Close {
        # "Abort playback window and ourself"
        n297 = event-data() -> ()  [unwired: 1 in, 4 out]
        n298 = invoke class="VI" method="FP.Close"(reference=w458) -> (reference out=w457:refnum<vi>)  [unwired: 2 in, 2 out]
        n299 = invoke class="VI" method="Abort VI"(reference=w457) -> (error out=w456:errorcluster)  [unwired: 2 in, 2 out]
        n300 = invoke class="VI" method="Abort VI"(error in=w456) -> ()  [unwired: 2 in, 3 out]
      }
      event User Event {
        n301 = event-data() -> ("IDs"=w465:cluster{"RPC field ID":u16, "Unique ID":u16}, "String"=w464:string)  [unwired: 1 in]
        n302 = Bundle("IDs"=w465, "String"=w464) -> (w463:T8)  [unwired: 1 in]
        n303 = call <vilib>:"Retrieve RPC Response.vi"("RPC Response"=w463) -> ("Output"=w461:string[][])  [unwired: 10 in]
        n304 = Build Array (concatenate)(w459, w461) -> (w460:string[][])
        n305 = local write "Command Params"(w460) -> ()
        n306 = local write "Cmd Status"("" ("Cmd Status")) -> ()
      }
      event "Tree": Double Click {
        n307 = event-data() -> ("PlatMods"=w471:T22, "Tag"=w468:string)  [unwired: 1 in]
        n308 = Unbundle(w471) -> ("Shift"=w470:bool)  [unwired: 4 out]
        n309 = String Subset(string=w468, length (rest)=1 ("length (rest)")) -> (substring=w467:string)  [unwired: 1 in]
        n310 = Not(x=w470) -> (.not. x?=w469:bool)
        n311 = case shown="\"/\"" w467 {
          tunnel: w468 -> [_ w474]
          tunnel: w469 -> [_ w473]
          frame Default {
          }
          frame "/" {
            n312 = call <vilib>:"NT Update Persistence.vi"("Persistence"=w473, "Name"=w474) -> ()  [unwired: 9 in, 1 out]
          }
        }
      }
    }
  }
  n313 = while {
    tunnel: w65 -> [w476]
    i -> [w479]
    stop <- FALSE stop-if-true
    n314 = Wait (ms)(milliseconds to wait=u32 100) -> ()  [unwired: 1 out]
    n315 = case shown="\"Playback\"" "Rec Mode" {
      tunnel: w479 -> [_ _ w494]
      tunnel: [u32 2829099 ("Base Color") u32 11141120 ("Target Color") w483] -> w475
      frame "Stop", Default {
        # "Reset the color, extra updates don't cost much"
      }
      frame "Record" {
      }
      frame "Playback" {
        # "Playback"
        n316 = Quotient & Remainder(x=w494, y=u32 50 ("milliseconds to wait")) -> (x-y*floor(x/y)=w490:u32)  [unwired: 1 out]
        n317 = Divide(x=w490, y=u32 50 ("milliseconds to wait")) -> (x/y=w487:dbl)
        n318 = Multiply(x=6.283185307179586, y=w487) -> (x*y=w492:dbl)
        n319 = Sine(x=w492) -> (sin(x)=w491:dbl)
        n320 = Absolute Value(x=w491) -> (abs(x)=w484:dbl)
        n321 = call "Interpolate RGB Color.vi"("Proportion"=w484, "Target Color"=u32 30976, "Base Color"=u32 2829099) -> ("Result Color"=w483:u32)  [unwired: 8 in]
      }
    }
    n322 = property class="Pane"(reference=w476, "PaneColor"=w475) -> ()  [unwired: 1 in, 2 out]
  }
  n323 = local write "Dashboard Tab"(T2."Drive" ("Dashboard Tab")) -> ()
  n324 = property on="On/Off" class="Bool (strict)"("Visible"=w36) -> ()  [unwired: 2 in, 2 out]
  n325 = property on="Motor" class="Clust (strict)"("Visible"=w36) -> ()  [unwired: 2 in, 2 out]
  n326 = property on="Progress" class="Clust (strict)"("Visible"=w36) -> ()  [unwired: 2 in, 2 out]
  n327 = property on="Test Ring" class="Ring (strict)"("Visible"=w36) -> ()  [unwired: 2 in, 2 out]
  n328 = property on="Rev/Fwd" class="Clust (strict)"("Visible"=w36) -> ()  [unwired: 2 in, 2 out]
  n329 = while {
    tunnel: u16 1741 ("timeout ms (25000)") -> [w496]
    stop <- FALSE stop-if-true
    n330 = TCP Create Listener(10:w496) -> (0:w495:errorcluster, 3:w497:refnum<k5>)  [unwired: 4 in, 1 out]
    n331 = case shown="No Error" w495 {
      selector: w495 -> [w499 _]
      tunnel: w497 -> [w500 _]
      frame No Error {
        n332 = while {
          tunnel: w500 -> [w503]
          tunnel: w499 -> [w502]
          stop <- FALSE stop-if-true
          n333 = TCP Wait On Listener(8:w502, 11:w503) -> (0:w504:errorcluster, 4:w505:refnum<k5>)  [unwired: 2 in, 3 out]
          n334 = local write "TCP"(w505) -> ()
          n335 = case shown="No Error" w504 {
            frame No Error {
            }
            frame Error {
              n336 = Wait (ms)(milliseconds to wait=u32 1000) -> ()  [unwired: 1 out]
            }
          }
        }
      }
      frame Error {
        n337 = Wait (ms)(milliseconds to wait=u32 1000) -> ()  [unwired: 1 out]
      }
    }
  }
  n338 = local write "Command Selection"(u16 0 ("milliseconds to wait")) -> ()
  n339 = local write "Command Params"(string[][] [] ("Command Params")) -> ()
  n340 = global write "WPI_DashboardLogging Global.vi" "Recording"(w59) -> ()
  n341 = local write "Rec Mode"(w59) -> ()
  n342 = call <vilib>:"NT Write String.vi"("String"="Select Auto", "Name"="Auto Selector") -> ()  [unwired: 9 in, 1 out]
